vi "Cluster Bundler Get Typedef Terminal.vi"(8 "error in (no error)":errorcluster, 11 "GObject in":refnum<vi>) -> (0 "error out":errorcluster, 3 "Terminal out":refnum<vi>)   [LabVIEW 2014]
doc: "Returns reference to Terminal where has to be connected Cluster which specify how to Bundle items."
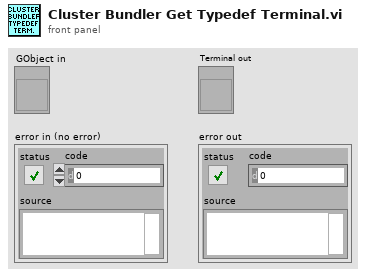
[diagram p1: front panel]
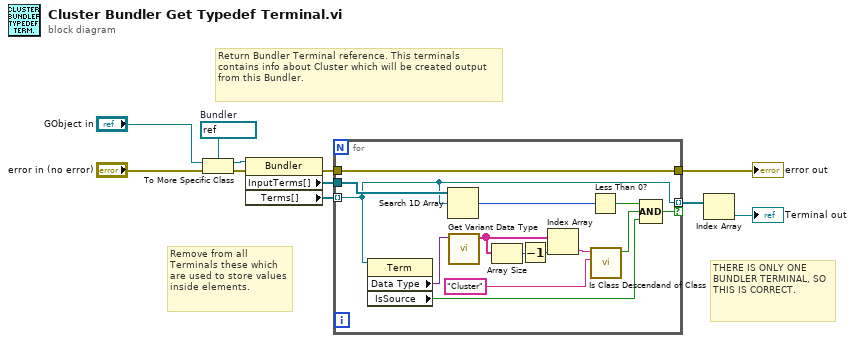
[diagram p0: block diagram]
diagram:
  w2 = refnum<vi> refnum  # Bundler
  # "THERE IS ONLY ONE BUNDLER TERMINAL, SO THIS IS CORRECT."
  # "Remove from all Terminals these which are used to store values inside elements."
  # "Return Bundler Terminal reference. This terminals contains info about Cluster which will be created output from this Bundler."
  n1 = To More Specific Class(target class=w2, reference="GObject in", error in="error in (no error)") -> (specific class reference=w3:refnum<vi>, error out=w4:errorcluster)
  n2 = property on="Property Node" class="Bundler"(reference=w3, error in=w4) -> (error out=w10:errorcluster, "InputTerms[]"=w6:refnum<vi>[], "Terms[]"=w5:refnum<vi>[])  [unwired: 1 out]
  n3 = for {
    tunnel: w5 -> [w21] mode=indexing
    tunnel: w6 -> [w25]
    tunnel: [w21] -> w7 mode=indexing if=w20
    tunnel: w10 -> [w18]
    tunnel: [w18] -> w11
    n4 = property class="Term"(reference=w21) -> ("Data Type"=w23:variant, "IsSource"=w19:bool)  [unwired: 1 in, 2 out]
    n5 = Search 1D Array(1D array=w25, element=w21) -> (index of element=w24:i32)  [unwired: 1 in]
    n6 = call "Get Variant Data Type.vi"("Variant in"=w23) -> ("Data Types[]"=w14:string[])  [unwired: 9 in, 1 out]
    n7 = Array Size(array=w14) -> (size(s)=w13:i32)
    n8 = Decrement(x=w13) -> (x-1=w12:i32)
    n9 = Index Array(array=w14, index=w12) -> (element=w15:string)
    n10 = Less Than 0?(x=w24) -> (x < 0?=w22:bool)
    n11 = call "Is Class Descendand of Class.vi"("Parent ClassName"="Cluster" ("x"), "ClassName"=w15) -> ("is Class descendant?"=w16:bool)  [unwired: 8 in, 1 out]
    n12 = Compound Arithmetic op=AND(w22, w16, w19) -> (w20:bool)
  }
  "error out" <- w11
  n13 = Index Array(array=w7) -> (element=→"Terminal out":refnum<vi>)  [unwired: 1 in]
